vi "Generate Unique Header.vi"(8 "error in":errorcluster, 11 "Single_Array in":refnum<class "Single_Array.lvclass">) -> (0 "error out":errorcluster, 2 "Header":string[](array[string]), 3 "Single_Array out":refnum<class "Single_Array.lvclass">)   [LabVIEW 2014, in "Base Data Class.lvlib" / "Single_Array.lvclass"]
uses:
  Single_Array.lvclass
  Single_Array.lvclass/Single_Array.ctl
  Data.lvclass
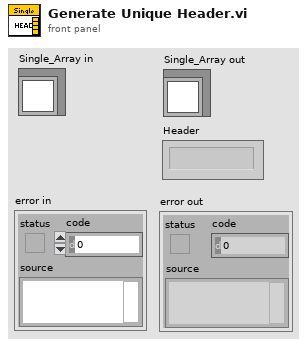
[diagram p1: front panel]
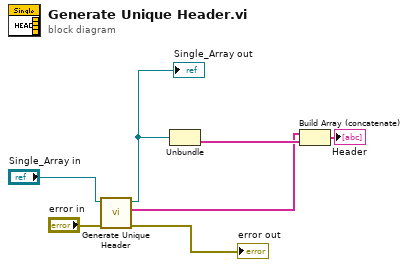
[diagram p0: block diagram]
diagram:
  n1 = call-parent "Generate Unique Header.vi"("error in"="error in", "Data in"="Single_Array in") -> ("error out"=→"error out":errorcluster, "Header"=w2:string[], "Data out"=w4:refnum<class "Single_Array.lvclass">)  [unwired: 7 in]
  "Single_Array out" <- w4
  n2 = Unbundle(w4) -> (w3:string[])  [unwired: 1 out]
  n3 = Build Array (concatenate)(w2, w3) -> (→"Header":string[])
